vi "Initialize.vi"(6 "optional":variant, 8 "error in (no error)":errorcluster, 11 "PriorityNode data":refnum<class "PriorityNode.lvclass">) -> (0 "error out":errorcluster, 3 "Node out":refnum<data-value>)   [LabVIEW 2009, in "PriorityNode.lvclass"]
uses:
  PriorityNode.lvclass
  Node/Node.lvclass
  Message/Message.lvclass
  LLNode/LLNode.lvclass
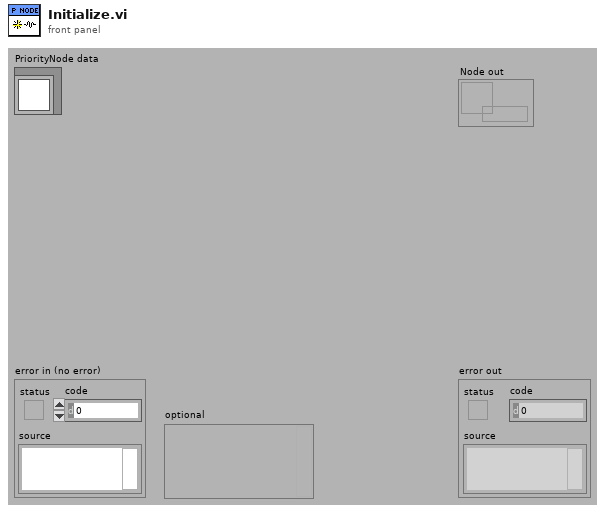
[diagram p1: front panel]
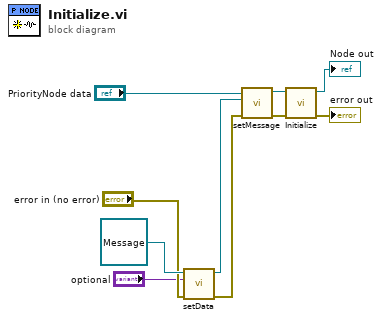
[diagram p0: block diagram]
diagram:
  n1 = call "setData.vi"("error in (no error)"="error in (no error)", "Data"="optional", "Message in"=refnum<class "Message.lvclass"> refnum ("Message.lvclass")) -> ("error out"=w7:errorcluster, "Message out"=w6:refnum<class "Message.lvclass">)  [unwired: 7 in]
  n2 = call "setMessage.vi"("error in (no error)"=w7, "Message.lvclass"=w6, "PriorityNode in"="PriorityNode data") -> ("error out"=w1:errorcluster, "PriorityNode out"=w2:refnum<class "PriorityNode.lvclass">)  [unwired: 7 in]
  n3 = call-parent "Initialize.vi"("error in (no error)"=w1, "LLNode data"=w2) -> ("error out"=→"error out":errorcluster, "Node out"=→"Node out":refnum<data-value>)  [unwired: 8 in]
